vi "GetDefaultClicks.vi"(8 "error in (no error)":errorcluster, 11 "MGI_MenuItem in":refnum<class "MGI_MenuItem.lvclass">) -> (0 "error out":errorcluster, 2 "Default Click Tags":string[](array[string]), 3 "MGI_MenuItem out":refnum<class "MGI_MenuItem.lvclass">)   [LabVIEW 2016, in "MGI_MenuItem.lvclass"]
doc: "Recursively searches its self and it's submenus to determin if there are any items that should be clicked by default.\n\nAuthored by Derek E. Trepanier\nsupport@mooregoodideas.com\nwww.mooregoodideas.com\n\nCopyright (c) 2012, Moore Good Ideas, Inc.\n\nAll rights reserved.\n\nRedistribution and use in source and binary forms, with or without modification, are permitted provided that the following conditions are met:\n\n * Redistributions of source code must retain the above copyright notice, this list of conditions and the following disclaimer.\n * Redistributions in binary form must reproduce the above copyright notice, this list of conditions and the following disclaimer in the documentation and/or other materials provided with the distribution.\n * Neither the name of Moore Good Ideas, Inc. nor the names of its contributors may be used to endorse or promote products derived from this software without specific prior written permission.\n\nTHIS SOFTWARE IS PROVIDED BY THE COPYRIGHT HOLDERS AND CONTRIBUTORS \"AS IS\" AND ANY EXPRESS OR IMPLIED WARRANTIES, INCLUDING, BUT NOT LIMITED TO, THE IMPLIED WARRANTIES OF MERCHANTABILITY AND FITNESS FOR A PARTICULAR PURPOSE ARE DISCLAIMED. IN NO EVENT SHALL THE COPYRIGHT OWNER OR CONTRIBUTORS BE LIABLE FOR ANY DIRECT, INDIRECT, INCIDENTAL, SPECIAL, EXEMPLARY, OR CONSEQUENTIAL DAMAGES (INCLUDING, BUT NOT LIMITED TO, PROCUREMENT OF SUBSTITUTE GOODS OR SERVICES; LOSS OF USE, DATA, OR PROFITS; OR BUSINESS INTERRUPTION) HOWEVER CAUSED AND ON ANY THEORY OF LIABILITY, WHETHER IN CONTRACT, STRICT LIABILITY, OR TORT (INCLUDING NEGLIGENCE OR OTHERWISE) ARISING IN ANY WAY OUT OF THE USE OF THIS SOFTWARE, EVEN IF ADVISED OF THE POSSIBILITY OF SUCH DAMAGE."
uses:
  <userlib>/_MGI/Menu Building/MenuItem/MGI_MenuItem.lvclass
  <userlib>/_MGI/Menu Building/MenuItem/MGI_MenuItem.lvclass/MGI_MenuItem.ctl
  <userlib>/_MGI/Menu Building/MenuItem/Read Sub-Menus.vi
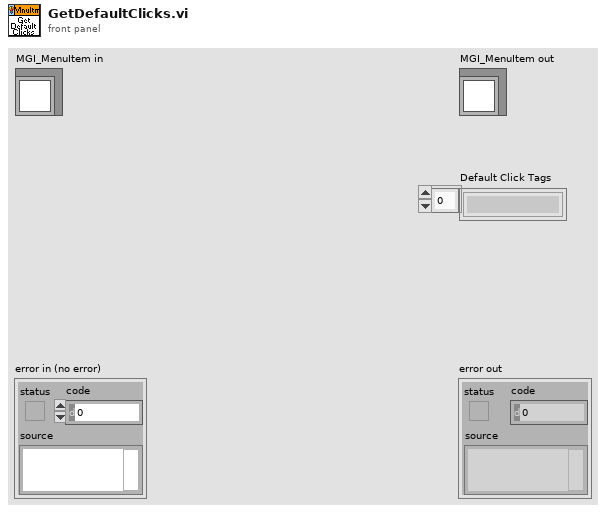
[diagram p1: front panel]
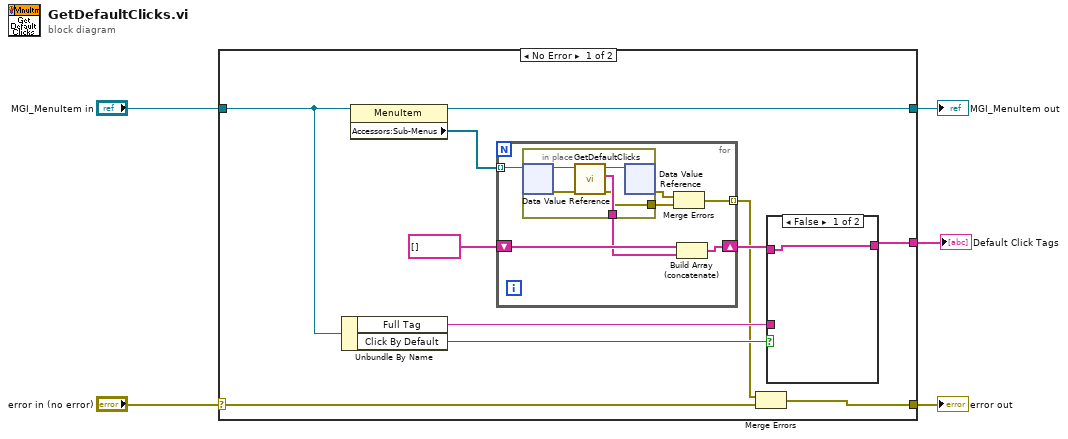
[diagram p0: block diagram]
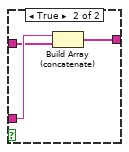
[diagram p2: hidden frame]
diagram:
  n1 = case shown="No Error" "error in (no error)" {
    selector: "error in (no error)" -> [w16 w34]
    tunnel: [w7 w34] -> w4
    tunnel: [w14 w33] -> w2
    tunnel: "MGI_MenuItem in" -> [w15 w33]
    tunnel: [w8 _] -> w1
    frame No Error {
      n2 = Unbundle By Name(w15) -> ("Full Tag"=w11:string, "Click By Default"=w12:bool)
      n3 = property class="MenuItem"(reference=w15) -> (reference out=w14:refnum<class "MGI_MenuItem.lvclass">, "Accessors:Sub-Menus"=w13:refnum<data-value>[])  [unwired: 1 in, 1 out]
      n4 = for {
        tunnel: w13 -> [w25] mode=indexing
        shift-right: [w26] -> w9
        shift-left: string[] [] ("Default Click Tags") -> [w27]
        tunnel: [w21] -> w6 mode=indexing
        n5 = in-place {
          in-place-border: [w29] -> w24
          in-place-border: [w28] -> w22
          n6 = in-place-dvr #1(w25) -> (w31:refnum<class "MGI_MenuItem.lvclass">, w30:errorcluster)
          n7 = call <userlib>:"GetDefaultClicks.vi"("error in (no error)"=w30, "MGI_MenuItem in"=w31) -> ("error out"=w28:errorcluster, "Default Click Tags"=w29:string[], "MGI_MenuItem out"=w32:refnum<class "MGI_MenuItem.lvclass">)  [unwired: 7 in]
          n8 = in-place-dvr #1(w32) -> (w23:errorcluster)  [unwired: 1 out]
        }
        n9 = Merge Errors(w23, w22) -> (w21:errorcluster)
        n10 = Build Array (concatenate)(w27, w24) -> (w26:string[])
      }
      n11 = Merge Errors(w6, w16) -> (w7:errorcluster)
      n12 = case shown="False" w12 {
        tunnel: w11 -> [_ w20]
        tunnel: w9 -> [w17 w19]
        tunnel: [w17 w18] -> w8
        frame False {
        }
        frame True {
          n13 = Build Array (concatenate)(w20, w19) -> (w18:string[])
        }
      }
    }
    frame Error {
    }
  }
  "error out" <- w4
  "MGI_MenuItem out" <- w2
  "Default Click Tags" <- w1
